vi "3.vi"() -> ()   [LabVIEW 2013]
panel:
  out "data out":string
  in  "Stop Button":bool
  out "error out":errorcluster
  in  "port":u16
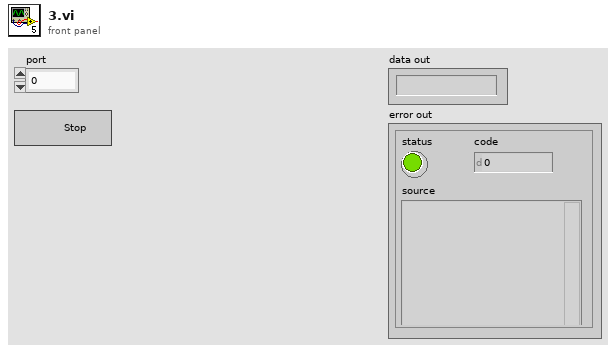
[diagram p1: front panel]
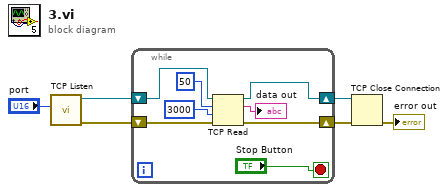
[diagram p0: block diagram]
diagram:
  n1 = call <vilib>:"TCP Listen.vi"("port"="port") -> ("error out"=w4:errorcluster, "connection ID"=w5:refnum<k5>)  [unwired: 6 in, 3 out]
  n2 = while {
    shift-right: [w9] -> w3
    shift-left: w5 -> [w14]
    shift-right: [w8] -> w2
    shift-left: w4 -> [w13]
    stop <- "Stop Button" stop-if-true
    n3 = TCP Read(connection ID=w14, bytes to read=50, error in (no error)=w13, 9:3000 ("timeout ms (25000)")) -> (connection ID out=w9:refnum<k5>, data out=→"data out":string, error out=w8:errorcluster)  [unwired: 1 in]
  }
  n4 = TCP Close Connection(connection ID=w3, error in (no error)=w2) -> (error out=→"error out":errorcluster)  [unwired: 1 in, 1 out]
